vi "ShowMapGlobalV2.2.vi"() -> ()   [LabVIEW 2014]
panel:
  in  "Show Map":cluster{"Color Box":u32, "String":string}[][](array[cluster])
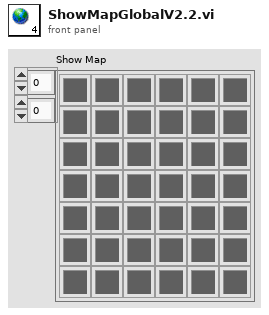
[diagram p1: front panel]
diagram:
